vi "Tester.vi"() -> ()   [LabVIEW 2018]
uses:
  State.ctl
  <vilib>/measure/NI_MABase.lvlib
panel:
  out "Waveform Chart":waveform(dbl)(graph)
  in  "Pause State machine":bool
  in  "Stop App":bool
  in  "Play State machine":bool
  out "State":T1
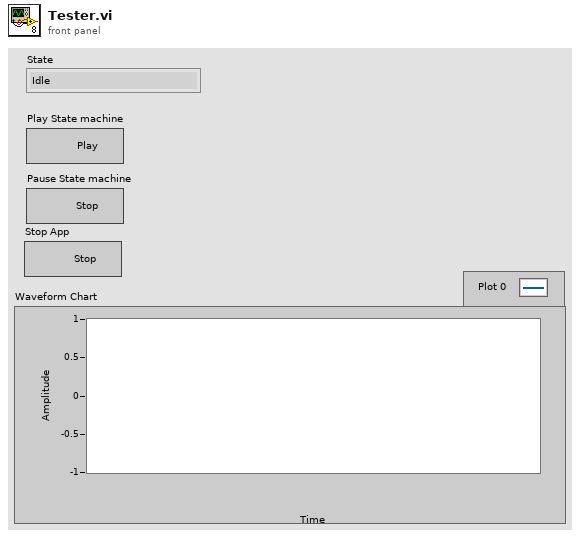
[diagram p1: front panel]
types:
  T1 = typedef "State.ctl" = enum16{"Idle", "Stop", "Play", "Init"}
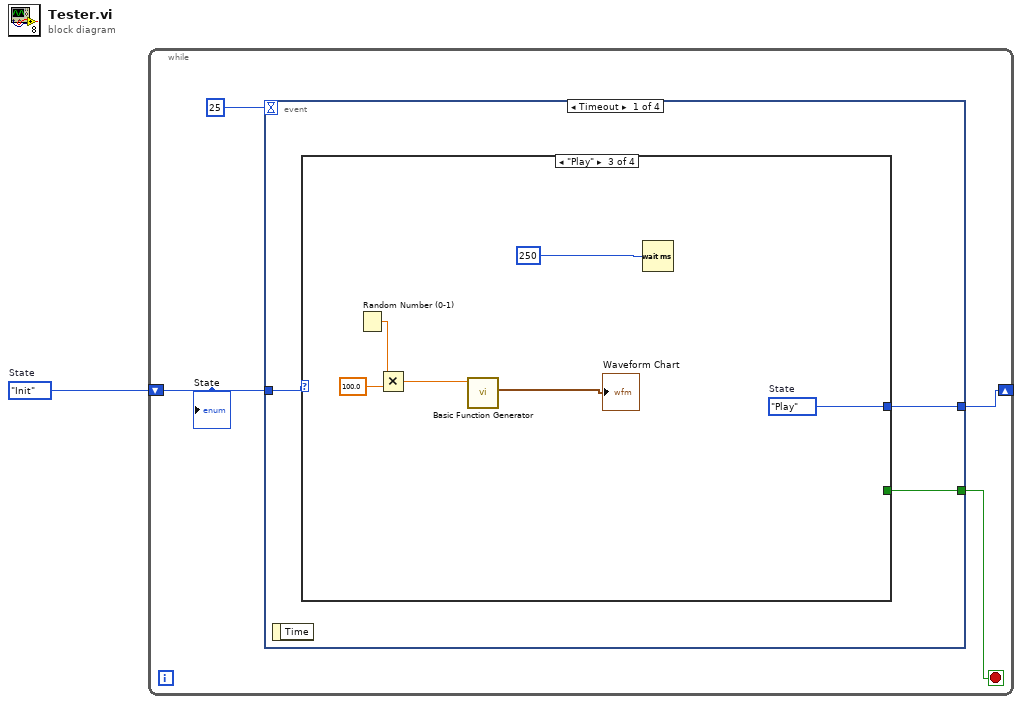
[diagram p0: block diagram]
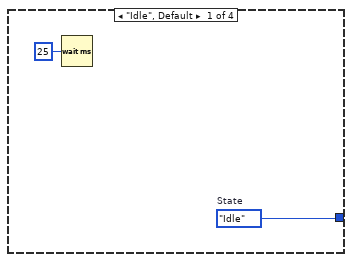
[diagram p2: hidden frame]
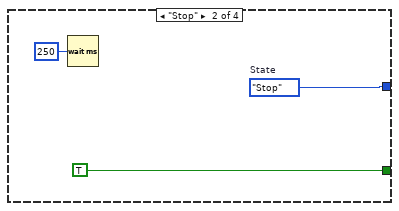
[diagram p3: hidden frame]
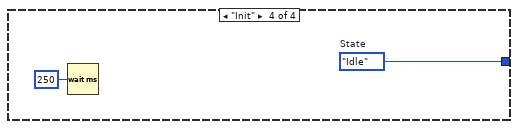
[diagram p4: hidden frame]
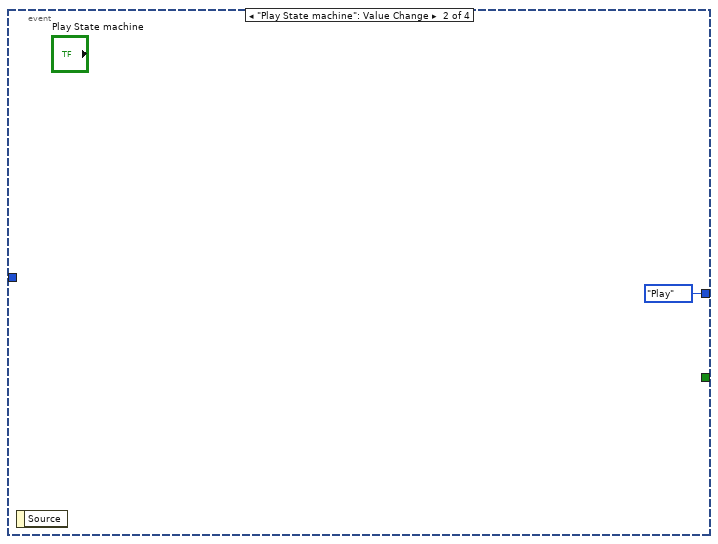
[diagram p5: hidden frame]
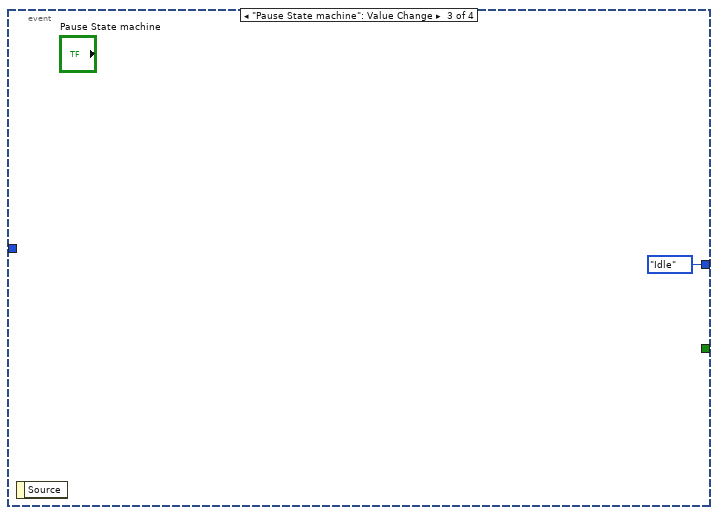
[diagram p6: hidden frame]
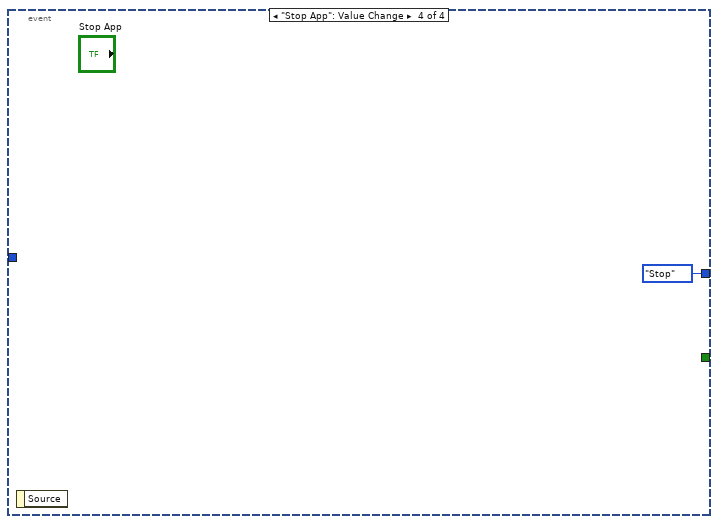
[diagram p7: hidden frame]
diagram:
  w1 = State."Init"  # State
  n1 = while {
    shift-right: [w4] -> _
    shift-left: w1 -> [w5]
    stop <- w3 stop-if-true
    n2 = event shown="[0] Timeout" {
      selector: _ -> [_ _ _ _]
      dyn-events: _ -> [_ _ _ _]
      timeout: 25 -> [_ _ _ _]
      tunnel: w5 -> [w8 _ _ _]
      tunnel: [w7 State."Play" ("State") State."Idle" ("State") State."Stop" ("State")] -> w4
      tunnel: [w6 _ _ _] -> w3
      event Timeout {
        n3 = event-data() -> ()  [unwired: 1 in, 1 out]
        n4 = case shown="\"Play\"" w8 {
          tunnel: [w10 w13 w19 w21] -> w7
          tunnel: [_ TRUE _ _] -> w6
          frame "Idle", Default {
            w10 = State."Idle"  # State
            n5 = Wait (ms)(milliseconds to wait=u32 25) -> ()  [unwired: 1 out]
          }
          frame "Stop" {
            w13 = State."Stop"  # State
            n6 = Wait (ms)(milliseconds to wait=u32 250) -> ()  [unwired: 1 out]
          }
          frame "Play" {
            w19 = State."Play"  # State
            n7 = Random Number (0-1)() -> (number: 0 to 1=w16:dbl)
            n8 = Multiply(x=w16, y=100.0) -> (x*y=w15:dbl)
            n9 = call <vilib>:"Basic Function Generator.vi"("frequency"=w15) -> ("signal out"=→"Waveform Chart":waveform(dbl))  [unwired: 8 in, 2 out]
            n10 = Wait (ms)(milliseconds to wait=u32 250) -> ()  [unwired: 1 out]
          }
          frame "Init" {
            w21 = State."Idle"  # State
            n11 = Wait (ms)(milliseconds to wait=u32 250) -> ()  [unwired: 1 out]
          }
        }
      }
      event "Play State machine": Value Change {
        n12 = event-data() -> ()  [unwired: 1 in, 1 out]
      }
      event "Pause State machine": Value Change {
        n13 = event-data() -> ()  [unwired: 1 in, 1 out]
      }
      event "Stop App": Value Change {
        n14 = event-data() -> ()  [unwired: 1 in, 1 out]
      }
    }
    "State" <- w5
  }
